vi "ADCP_UI_Continuous_Receiver_Log_File_Updater.vi"(8 "error in (no error)":errorcluster, 11 "ADCU_GUI References":T1) -> ()   [LabVIEW 2017]
uses:
  Controls/ADCP_UI/ADCP_UI_Parameters.ctl
  Controls/ADCP_UI/ADCP_UI_Queues.ctl
  Controls/ADCP_UI/ADCP_UI_Continuous_Receiver_States.ctl
  Controls/ADCP_UI/ADCP_Queue_Receive_Log_Queue_Element.ctl
  Controls/Packet/Packet.ctl
  Controls/Packet/Packet_Direction.ctl
  Controls/Packet/Packet_Type.ctl
  Controls/Packet/Packet_Priority.ctl
  Controls/Data Packets/Data_Packet.ctl
  Controls/Data Packets/Parameter.ctl
  Controls/Data Packets/Parameter_Data_Type.ctl
  Controls/Data Packets/Data_Packet_Transmit_Mode.ctl
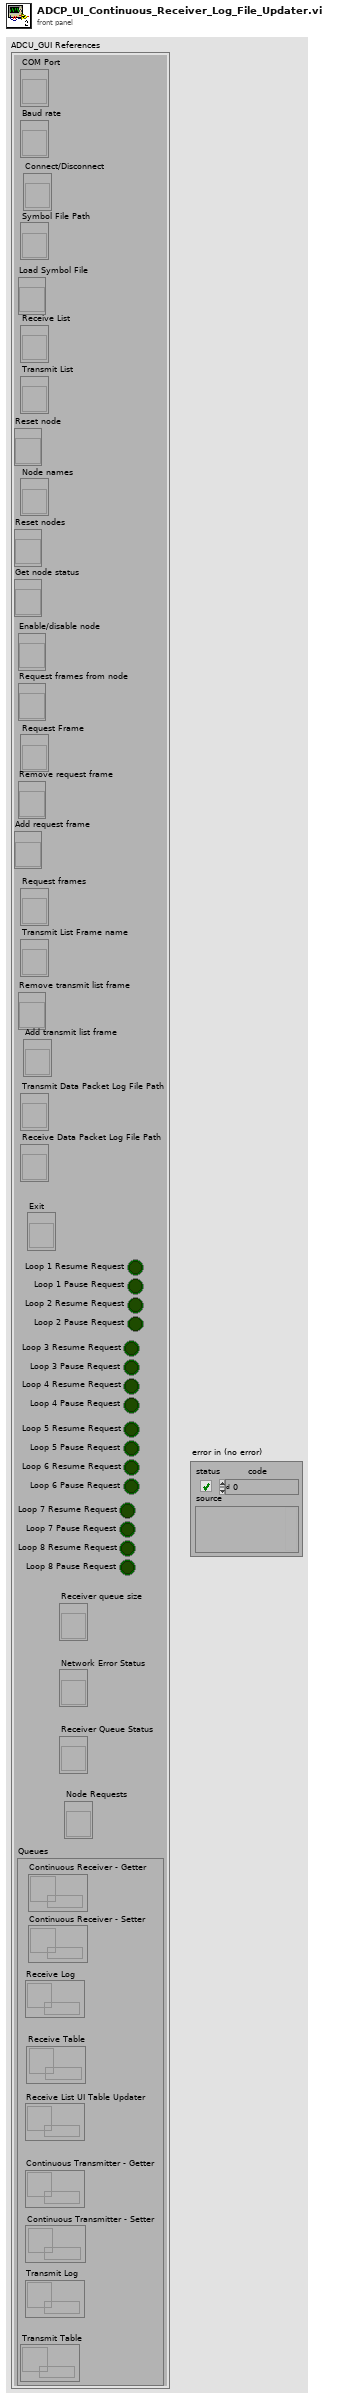
[diagram p1: front panel]
types:
  T1 = typedef "ADCP_UI_Parameters.ctl" = cluster{"COM Port":refnum<vi>, "Baud rate":refnum<vi>, "Symbol File Path":refnum<vi>, "Receive List":refnum<vi>, "Transmit List":refnum<vi>, "Node names":refnum<vi>, "Request Frame":refnum<vi>, "Request frames":refnum<vi>, "Transmit List Frame name":refnum<vi>, "Transmit Data Packet Log File Path":refnum<vi>, "Receive Data Packet Log File Path":refnum<vi>, "Loop 1 Resume Request":bool, "Loop 1 Pause Request":bool, "Loop 2 Resume Request":bool, "Loop 2 Pause Request":bool, "Loop 3 Resume Request":bool, "Loop 3 Pause Request":bool, "Loop 4 Resume Request":bool, "Loop 4 Pause Request":bool, "Loop 5 Resume Request":bool, "Loop 5 Pause Request":bool, "Loop 6 Resume Request":bool, "Loop 6 Pause Request":bool, "Loop 7 Resume Request":bool, "Loop 7 Pause Request":bool, "Loop 8 Resume Request":bool, "Loop 8 Pause Request":bool, "Exit":refnum<vi>, "Connect/Disconnect":refnum<vi>, "Load Symbol File":refnum<vi>, "Reset node":refnum<vi>, "Reset nodes":refnum<vi>, "Get node status":refnum<vi>, "Enable/disable node":refnum<vi>, "Request frames from node":refnum<vi>, "Remove request frame":refnum<vi>, "Add request frame":refnum<vi>, "Remove transmit list frame":refnum<vi>, "Add transmit list frame":refnum<vi>, "Receiver queue size":refnum<vi>, "Network Error Status":refnum<vi>, "Receiver Queue Status":refnum<vi>, "Node Requests":refnum<vi>, "Queues":T2}
  T2 = typedef "ADCP_UI_Queues.ctl" = cluster{"Continuous Receiver - Getter":refnum<queue>, "Continuous Receiver - Setter":refnum<queue>, "Receive Log":refnum<queue>, "Receive Table":refnum<queue>, "Receive List UI Table Updater":refnum<queue>, "Continuous Transmitter - Getter":refnum<queue>, "Continuous Transmitter - Setter":refnum<queue>, "Transmit Log":refnum<queue>, "Transmit Table":refnum<queue>}
  T3 = typedef "ADCP_Queue_Receive_Log_Queue_Element.ctl" = cluster{"Packet":T4, "Receive Time (ms)":u64, "Count":i32, "Receive Time Interval (ms) ":u64}
  T4 = typedef "Packet.ctl" = cluster{"Raw Bytes":u8[], "Checksum":bool, "Direction":T5, "Processed Bytes":u8[], "Node ID":u8, "Packet type":T6, "Frame Data":u32, "Priority":T7, "Frame ID":u8}
  T5 = typedef "Packet_Direction.ctl" = enum16{"Transmit", "Receive", "Bidirectional"}
  T6 = typedef "Packet_Type.ctl" = enum16{"Data", "Connection Management", "Remote Request", "Error/Status"}
  T7 = typedef "Packet_Priority.ctl" = enum16{"LOW", "HIGH"}
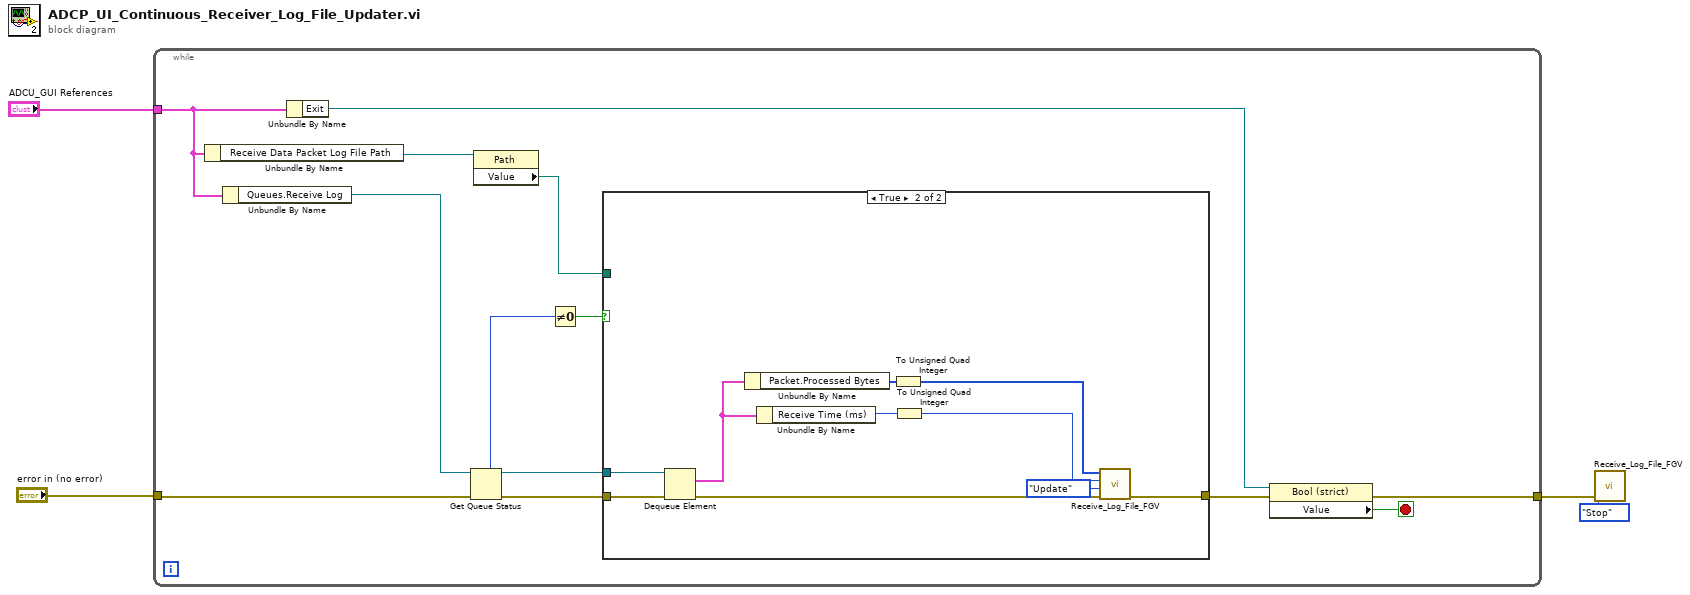
[diagram p0: block diagram]
diagram:
  n1 = while {
    tunnel: "error in (no error)" -> [w17]
    tunnel: "ADCU_GUI References" -> [w8]
    tunnel: [w9] -> w2
    stop <- w10 stop-if-true
    n2 = Unbundle By Name(w8) -> ("Receive Data Packet Log File Path"=w7:refnum<vi>)
    n3 = Unbundle By Name(w8) -> ("Queues.Receive Log"=w16:refnum<queue>)
    n4 = Unbundle By Name(w8) -> ("Exit"=w11:refnum<vi>)
    n5 = Get Queue Status(queue=w16, error in (no error)=w17) -> (queue out=w5:refnum<queue>, error out=w14:errorcluster, # elements in queue=w15:i32)  [unwired: 1 in, 5 out]
    n6 = property class="Path"(reference=w7) -> ("Value"=w6:path)  [unwired: 1 in, 2 out]
    n7 = Not Equal To 0?(x=w15) -> (x != 0?=w13:bool)
    n8 = case shown="True" w13 {
      tunnel: w14 -> [w18 w28]
      tunnel: [w18 w22] -> w12
      tunnel: w6 -> [_ _]
      tunnel: w5 -> [_ w27]
      frame False {
      }
      frame True {
        n9 = Dequeue Element(queue=w27, error in (no error)=w28) -> (element=w25:T3, error out=w23:errorcluster)  [unwired: 1 in, 2 out]
        n10 = Unbundle By Name(w25) -> ("Packet.Processed Bytes"=w26:u8[])
        n11 = Unbundle By Name(w25) -> ("Receive Time (ms)"=w24:u64)
        n12 = To Unsigned Quad Integer(1:w26) -> (0:w21:u64[])
        n13 = To Unsigned Quad Integer(1:w24) -> (0:w20:u64)
        n14 = call "Receive_Log_File_FGV.vi"("error in (no error)"=w23, "Command"=enum16{"Initialize", "Update", "Stop"}."Update", "Time (ms)"=w20, "Processed bytes"=w21) -> ("error out"=w22:errorcluster)  [unwired: 6 in, 1 out]
      }
    }
    n15 = property class="Bool (strict)"(reference=w11, error in=w12) -> (error out=w9:errorcluster, "Value"=w10:bool)  [unwired: 1 out]
  }
  n16 = call "Receive_Log_File_FGV.vi"("error in (no error)"=w2, "Command"=enum16{"Initialize", "Update", "Stop"}."Stop") -> ()  [unwired: 8 in, 2 out]
